vi "Save Image To File (UTF-8).vi"(7 "Save Format":T1, 8 "error in (no error)":errorcluster, 10 "Image":T2, 11 "Path In":string) -> (0 "error out":errorcluster, 3 "Path Out":string)   [LabVIEW 2020, in "G-Image.lvlib"]
doc: "Saves an image in the selected format to disk."
uses:
  G-Image.lvlib
  <vilib>/picture/picture.llb/imagedata.ctl
  Controls/Image Save Format.ctl
  Private/Result To Error.vi
  Private/ARGB To RGBA.vi
  <vilib>/Utility/error.llb/Error Cluster From Error Code.vi
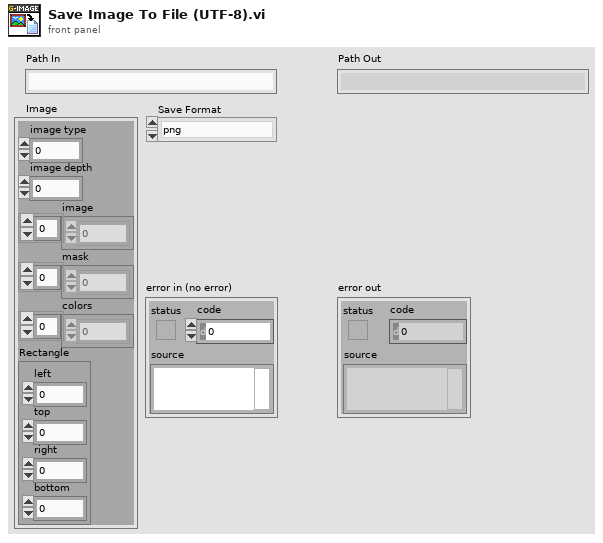
[diagram p1: front panel]
types:
  T1 = typedef "G-Image.lvlib/Image Save Format.ctl" = enum16{"png", "jpg", "bmp", "gif", "tga"}
  T2 = typedef "imagedata.ctl" = cluster{"image type":i32, "image depth":i32, "image":u8[], "mask":u8[], "colors":u32[], "Rectangle":cluster{"left":i16, "top":i16, "right":i16, "bottom":i16}}
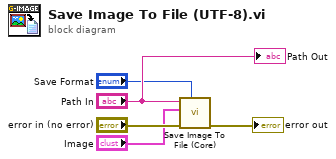
[diagram p0: block diagram]
diagram:
  n1 = call "Save Image To File (Core).vi"("Save Format"="Save Format", "error in (no error)"="error in (no error)", "Image"="Image", "Path In"="Path In") -> ("error out"=→"error out":errorcluster)  [unwired: 6 in, 1 out]
  "Path Out" <- "Path In"
